vi "Disconnect.vi"(8 "error in":errorcluster, 11 "Kronos in":refnum<class "Kronos.lvclass">) -> (0 "error out":errorcluster, 3 "Kronos out":refnum<class "Kronos.lvclass">)   [LabVIEW 2018, in "Kronos.lvlib" / "Kronos.lvclass"]
uses:
  Kronos.lvclass
  builds/Laser.lvlibp/Laser.lvclass
  C:/Users/Ron.Dexter.LUMINARTECH/Desktop/builds/Laser.lvlibp/Laser.lvclass
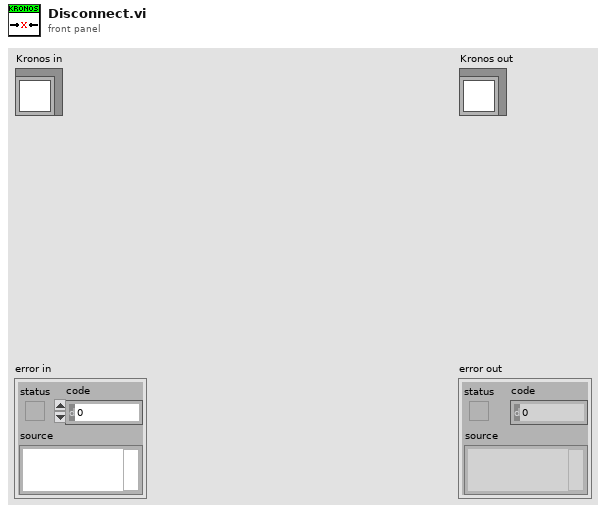
[diagram p1: front panel]
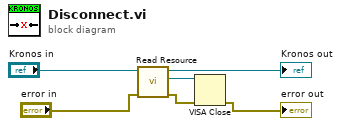
[diagram p0: block diagram]
diagram:
  n1 = call "Read Resource.vi"("error in (no error)"="error in", "Laser in"="Kronos in") -> ("error out"=w2:errorcluster, "Resource"=w3:refnum<visa-resource-name>, "Laser out"=→"Kronos out":refnum<class "Kronos.lvclass">)  [unwired: 7 in]
  n2 = VISA Close(VISA resource name=w3, error in (no error)=w2) -> (error out=→"error out":errorcluster)
